vi "RDS Child Receive Message.vi"(8 "error in (no error)":errorcluster, 10 "RDS Message":refnum<class "RDS Message.lvclass">, 11 "LSR Instrument in":refnum<class "LSR Instrument.lvclass">) -> (0 "error out":errorcluster, 3 "LSR Instrument out":refnum<class "LSR Instrument.lvclass">)   [LabVIEW 2015, in "LSR Instrument.lvlib" / "LSR Instrument.lvclass"]
uses:
  LSR Instrument.lvclass
  Libraries/RDS Framework/RDS Message Class/RDS Message.lvclass
  Libraries/RDS Framework/RDS Message Class/RDS Message.lvclass/RDS Message.ctl
  Libraries/RDS Child Messages/State Sample Message/State Sample Message.lvclass
  LSR Instrument.lvclass/LSR Instrument.ctl
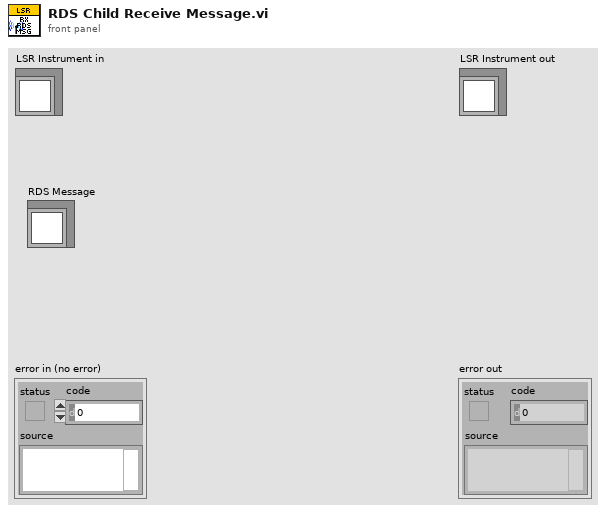
[diagram p1: front panel]
types:
  T1 = typedef "RDS Child Messages.lvlib/RDS Message ID.ctl" = enum16{"RDS Hello World", "String Message", "AIP_Status", "AIP_Command", "GPS_Data", "MCB_Command", "MCB_Status", "Compass_Data", "Depth_Data", "Battery_Data", "Contoller_State", "Set_Mag_Dev", "BTB_Shutdown", "State_Sample_Request", "State_Sample", "PID_Gains_Set", "Helm_Limiter_Set", "Helm_Heading_Command", "Helm_Steering_Command", "Helm_Status", "Controller_Message", "AIP_Set_Min_Depth", "Mission_Controller_State", "Mission_Upload", "Mission_Set_Op_and_Run", "Mission_Settings_Set"}
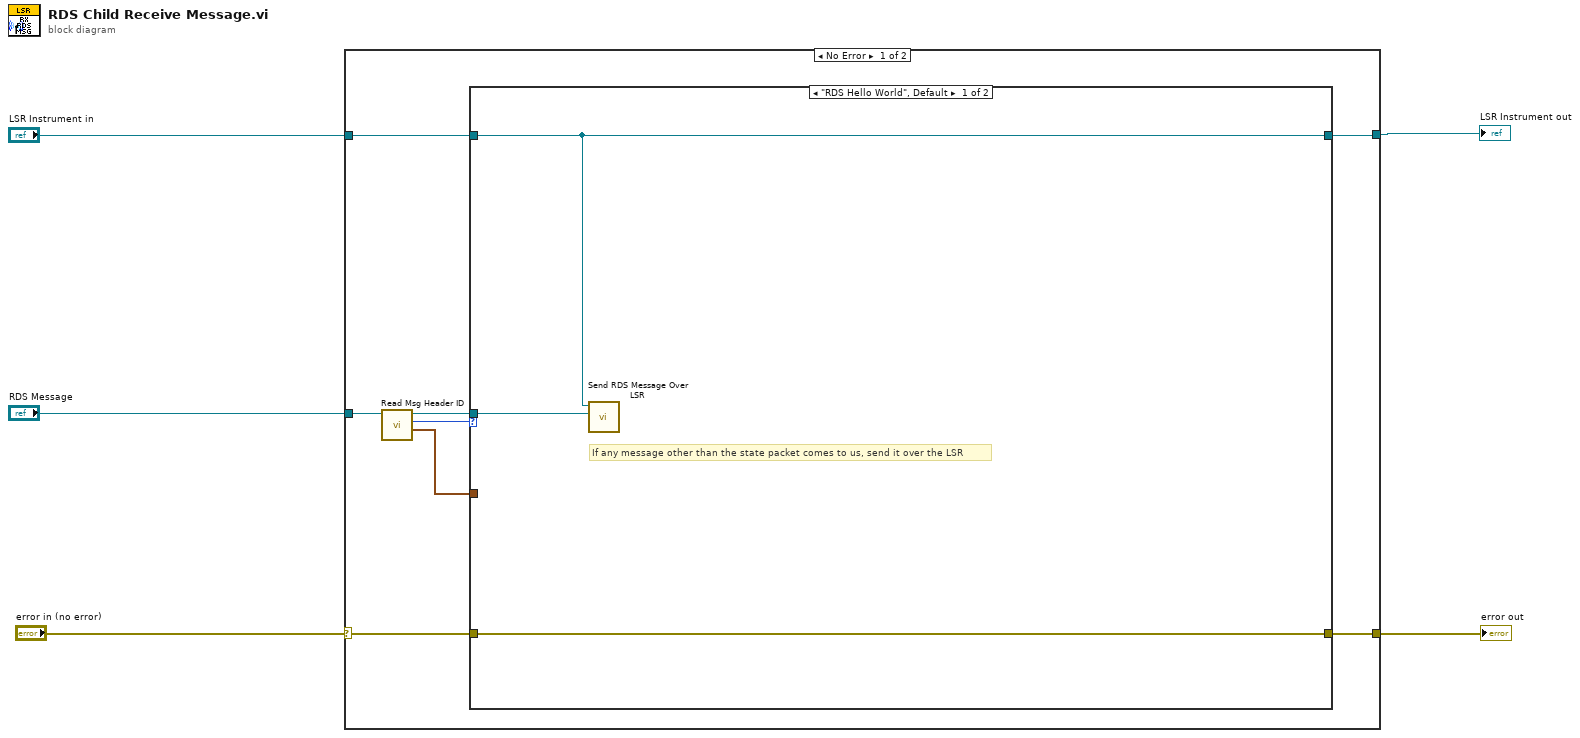
[diagram p0: block diagram]
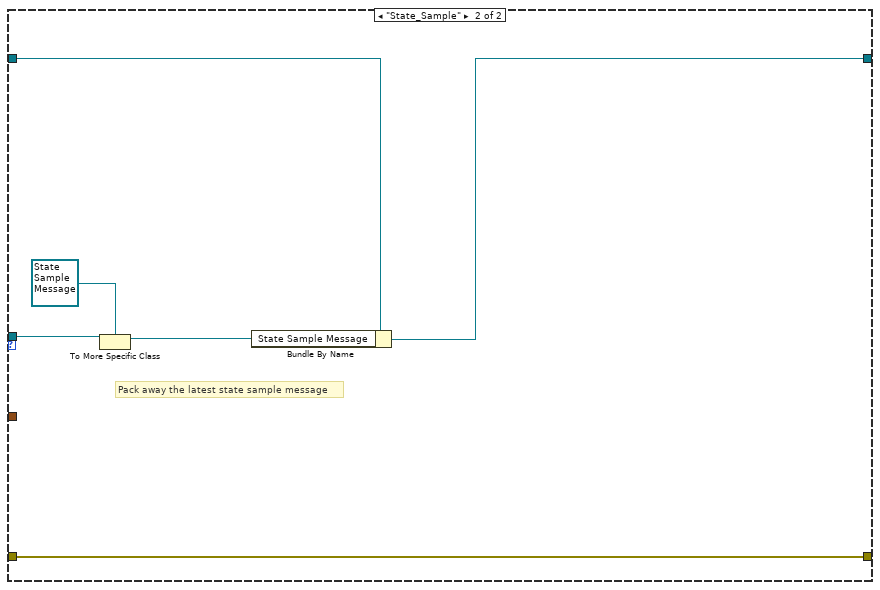
[diagram p2: hidden frame]
diagram:
  n1 = case shown="No Error" "error in (no error)" {
    selector: "error in (no error)" -> [w9 w23]
    tunnel: "RDS Message" -> [w13 _]
    tunnel: "LSR Instrument in" -> [w7 w24]
    tunnel: [w8 w24] -> w4
    tunnel: [w10 w23] -> w1
    frame No Error {
      n2 = call "Read Msg Header ID.vi"("RDS Message in"=w13) -> ("Time Stamp"=w6:timestamp, "Msg ID"=w12:T1, "RDS Message out"=w11:refnum<class "RDS Message.lvclass">)  [unwired: 6 in, 2 out]
      n3 = case shown="\"RDS Hello World\", Default" w12 {
        tunnel: w11 -> [w14 w21]
        tunnel: [w16 w22] -> w10
        tunnel: w9 -> [w16 w22]
        tunnel: w7 -> [w15 w19]
        tunnel: [w15 w18] -> w8
        tunnel: w6 -> [_ _]
        frame "RDS Hello World", Default {
          # "If any message other than the state packet comes to us, send it over the LSR"
          n4 = call "Send RDS Message Over LSR.vi"("RDS Child Message"=w14, "LSR Instrument in"=w15) -> ()  [unwired: 8 in, 2 out]
        }
        frame "State_Sample" {
          # "Pack away the latest state sample message"
          n5 = To More Specific Class(target class=refnum<class "State Sample Message.lvclass"> refnum ("RDS Child Messages.lvlib:State Sample Message.lvclass"), reference=w21) -> (specific class reference=w17:refnum<class "State Sample Message.lvclass">)  [unwired: 1 in, 1 out]
          n6 = Bundle By Name(cluster=w19, "State Sample Message"=w17) -> (w18:refnum<class "LSR Instrument.lvclass">)
        }
      }
    }
    frame Error {
    }
  }
  "error out" <- w1
  "LSR Instrument out" <- w4
